vi "CollectData.vi"(8 "error in (no error)":errorcluster, 11 "ArduinoDAC in":refnum<class "ArduinoDAC.lvclass">) -> (0 "error out":errorcluster, 3 "ArduinoDAC out":refnum<class "ArduinoDAC.lvclass">)   [LabVIEW 2013, in "ArduinoDAC.lvclass"]
uses:
  ArduinoDAC.lvclass
  Device/Device.lvclass
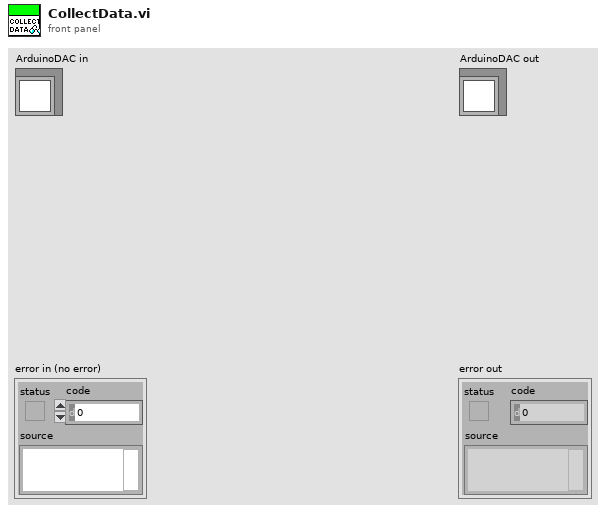
[diagram p1: front panel]
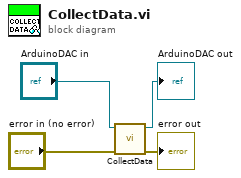
[diagram p0: block diagram]
diagram:
  n1 = call-parent "CollectData.vi"("error in (no error)"="error in (no error)", "Device in"="ArduinoDAC in") -> ("error out"=→"error out":errorcluster, "Device out"=→"ArduinoDAC out":refnum<class "ArduinoDAC.lvclass">)  [unwired: 8 in]
